vi "MUSIQCTrapControlNoStalling.vi"() -> ()   [LabVIEW 2012]
uses:
  <vilib>/DAQmx/read.llb/DAQmx Read (Counter U32 1Chan 1Samp).vi
  <vilib>/DAQmx/read.llb/DAQmx Read (Counter 1D U32 1Chan NSamp).vi
  <vilib>/DAQmx/create/channels.llb/DAQmx Create Channel (CO-Pulse Generation-Frequency).vi
  <vilib>/DAQmx/configure/timing.llb/DAQmx Timing (Implicit).vi
  <vilib>/DAQmx/create/channels.llb/DAQmx Create Channel (CI-Count Edges).vi
  <vilib>/DAQmx/configure/timing.llb/DAQmx Timing (Sample Clock).vi
  <vilib>/Analysis/baseanly.llb/Mean (DBL).vi
  <vilib>/DAQmx/miscellaneous.llb/DAQmx Fill In Error Info.vi
  <resource>/objmgr/daqmx.rc
  <vilib>/Analysis/NI_AALBase.lvlib
panel:
  in  "UV firing rate 2":dbl=2.0
  out "mean":i32
  in  "X window size":dbl=5.0
  out "Sample Rate":dbl
  out "PMT Counts 2":cluster{i32, u32}(graph)
  in  "Measure Background":bool
  in  "Pockel":bool=TRUE
  in  "Dump Frequency":dbl
  in  "AutoDump":bool
  out "Auto Loading Elapsed Time":dbl
  out "Loading Start Time":timestamp=timestamp(3525114376.279 s since 1904-01-01)
  in  "UV":bool
  in  "1762":bool
  in  "455 LED":bool
  in  "399 Yb Ionizer":bool
  in  "Oven":bool
  in  "Orange":bool=TRUE
  in  "Sample Time":dbl=0.02 format="%0.2f"
  in  "Threshold":u32
  in  "Auto Load":bool
  in  "RF":bool
  in  "Blue":bool=TRUE
  in  "Red":bool=TRUE
  in  "Samples per averaging\nblock red":i32=20 min=1 step=1
  in  "stop":bool
  out "PMT Counts":cluster{i32, u32}(graph)
  # "Trap 2"
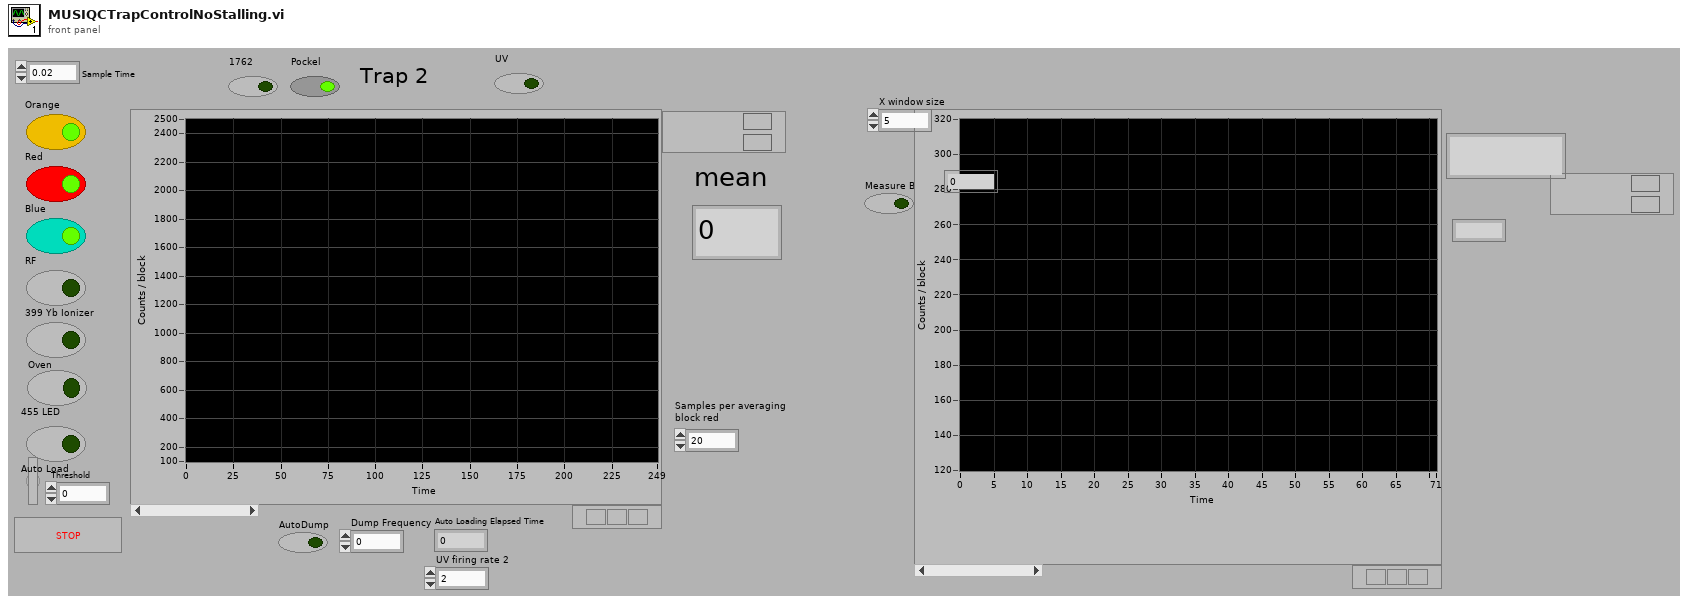
[diagram p1: front panel]
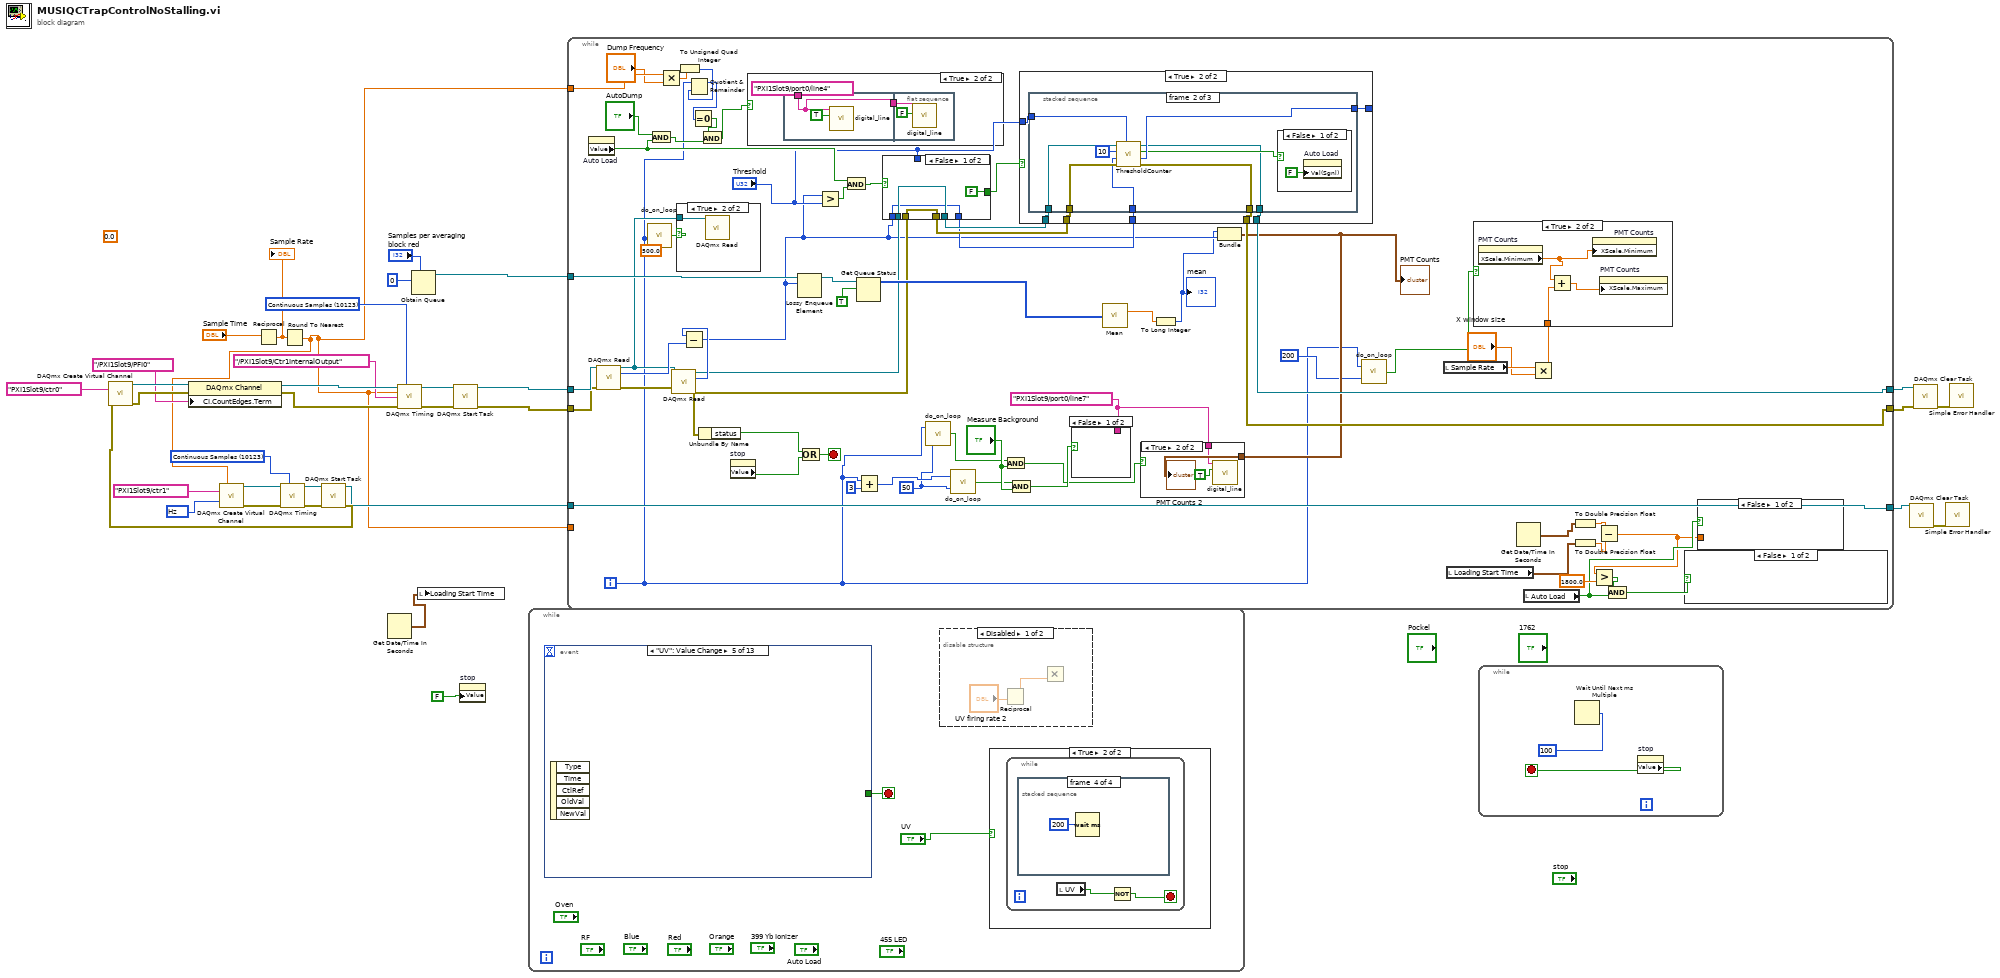
[diagram p0: block diagram]
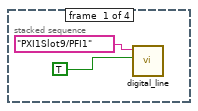
[diagram p3: hidden frame]
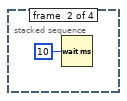
[diagram p4: hidden frame]
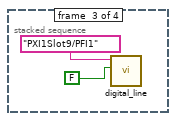
[diagram p5: hidden frame]
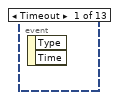
[diagram p7: hidden frame]
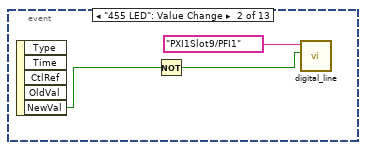
[diagram p8: hidden frame]
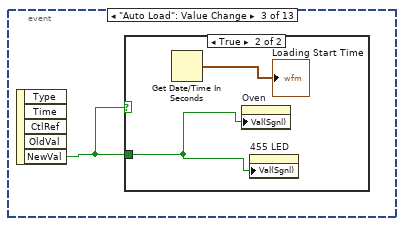
[diagram p9: hidden frame]
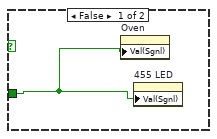
[diagram p10: hidden frame]
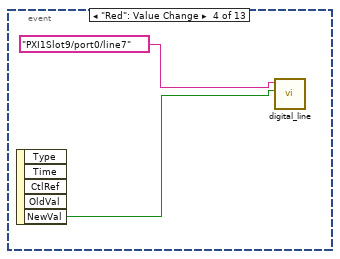
[diagram p11: hidden frame]
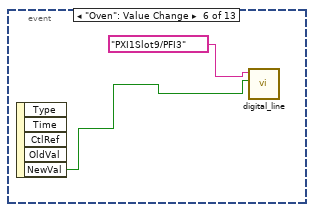
[diagram p12: hidden frame]
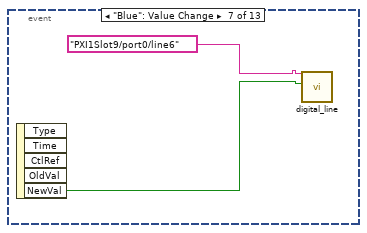
[diagram p13: hidden frame]
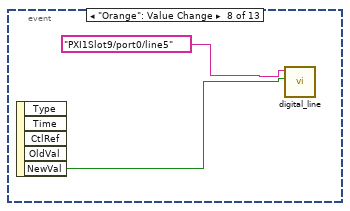
[diagram p14: hidden frame]
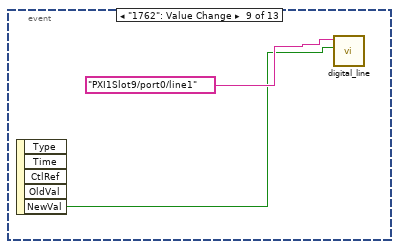
[diagram p15: hidden frame]
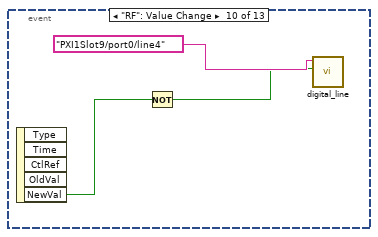
[diagram p16: hidden frame]
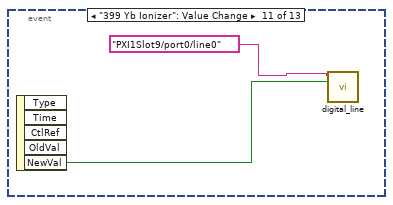
[diagram p17: hidden frame]
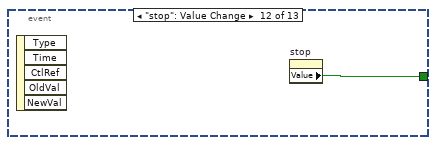
[diagram p18: hidden frame]
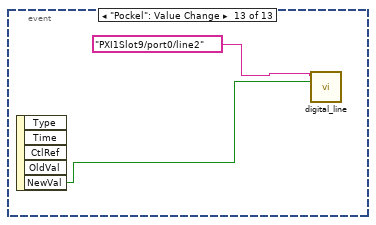
[diagram p19: hidden frame]
diagram:
  (unwired) 0.0 ("x")
  w5 = 10123 items=["Finite Samples"=10178, "Continuous Samples"=10123, "Hardware Timed Single Point"=12522] ("sample mode")
  w12 = 10373 items=["Hz"=10373] ("units")
  w18 = 10123 items=["Finite Samples"=10178, "Continuous Samples"=10123, "Hardware Timed Single Point"=12522] ("sample mode")
  n1 = Reciprocal(x="Sample Time") -> (1/x=w3:dbl)
  "Sample Rate" <- w3
  n2 = Round To Nearest(number=w3) -> (nearest integer value=w2:dbl)
  n3 = call-poly <vilib>:"DAQmx Create Virtual Channel.vi"("frequency"=w2, "counter"=tag "PXI1Slot9/ctr1", "units"=w12) -> ("task out"=w9:refnum<k21>, "error out"=w8:errorcluster)  [unwired: 11 in]
  n4 = call-poly <vilib>:"DAQmx Timing.vi"("task/channels in"=w9, "sample mode"=w5, "error in"=w8) -> ("task out"=w7:refnum<k21>, "error out"=w6:errorcluster)  [unwired: 11 in]
  n5 = call <vilib>:"DAQmx Start Task.vi"("task/channels in"=w7, "error in"=w6) -> ("task out"=w15:refnum<k21>, "error out"=w16:errorcluster)  [unwired: 12 in]
  n6 = call-poly <vilib>:"DAQmx Create Virtual Channel.vi"("counter"=tag "PXI1Slot9/ctr0", "error in"=w16) -> ("task out"=w26:refnum<k21>, "error out"=w25:errorcluster)  [unwired: 12 in]
  n7 = property class="DAQmx Channel"(reference=w26, error in=w25, "CI.CountEdges.Term"=tag "/PXI1Slot9/PFI0") -> (reference out=w28:refnum<k21>, error out=w27:errorcluster)
  n8 = Get Date/Time In Seconds() -> (seconds since 1Jan1904=w4:timestamp)
  n9 = call-poly <vilib>:"DAQmx Timing.vi"("task/channels in"=w28, "sample mode"=w18, "rate"=w2, "source"=tag "/PXI1Slot9/Ctr1InternalOutput", "error in"=w27) -> ("task out"=w33:refnum<k21>, "error out"=w32:errorcluster)  [unwired: 9 in]
  n10 = Obtain Queue(max queue size (-1, unlimited)="Samples per averaging\nblock red", element data type=u32 0) -> (queue out=w21:refnum<queue>)  [unwired: 3 in, 2 out]
  n11 = local write "Loading Start Time"(w4) -> ()
  n12 = call <vilib>:"DAQmx Start Task.vi"("task/channels in"=w33, "error in"=w32) -> ("task out"=w29:refnum<k21>, "error out"=w11:errorcluster)  [unwired: 12 in]
  n13 = property on="stop" class="Bool (strict)"("Value"=FALSE ("stop")) -> ()  [unwired: 2 in, 2 out]
  n14 = while {
    stop <- w36 stop-if-true
    n15 = event shown="[4] \"UV\": Value Change" {
      selector: _ -> [_ _ _ _ _ _ _ _ _ _ _ _ _]
      dyn-events: _ -> [_ _ _ _ _ _ _ _ _ _ _ _ _]
      timeout: _ -> [_ _ _ _ _ _ _ _ _ _ _ _ _]
      tunnel: [_ _ _ _ _ _ _ _ _ _ _ w69 _] -> w36
      event Timeout {
        n16 = event-data() -> ()  [unwired: 1 in, 2 out]
      }
      event "455 LED": Value Change {
        n17 = event-data() -> ("NewVal"=w49:bool)  [unwired: 1 in, 4 out]
        n18 = Not(x=w49) -> (.not. x?=w47:bool)
        n19 = call "digital_line.vi"("Boolean"=w47, "lines"=tag "PXI1Slot9/PFI1") -> ()  [unwired: 5 in, 1 out]
      }
      event "Auto Load": Value Change {
        n20 = event-data() -> ("NewVal"=w50:bool)  [unwired: 1 in, 4 out]
        n21 = case shown="True" w50 {
          tunnel: w50 -> [w51 w52]
          frame False {
            n22 = property on="Oven" class="Bool (strict)"("Val(Sgnl)"=w51) -> ()  [unwired: 2 in, 2 out]
            n23 = property on="455 LED" class="Bool (strict)"("Val(Sgnl)"=w51) -> ()  [unwired: 2 in, 2 out]
          }
          frame True {
            n24 = Get Date/Time In Seconds() -> (seconds since 1Jan1904=→"Loading Start Time":timestamp)
            n25 = property on="Oven" class="Bool (strict)"("Val(Sgnl)"=w52) -> ()  [unwired: 2 in, 2 out]
            n26 = property on="455 LED" class="Bool (strict)"("Val(Sgnl)"=w52) -> ()  [unwired: 2 in, 2 out]
          }
        }
      }
      event "Red": Value Change {
        n27 = event-data() -> ("NewVal"=w54:bool)  [unwired: 1 in, 4 out]
        n28 = call "digital_line.vi"("Boolean"=w54, "lines"=tag "PXI1Slot9/port0/line7") -> ()  [unwired: 5 in, 1 out]
      }
      event "UV": Value Change {
        n29 = event-data() -> ()  [unwired: 1 in, 5 out]
      }
      event "Oven": Value Change {
        n30 = event-data() -> ("NewVal"=w56:bool)  [unwired: 1 in, 4 out]
        n31 = call "digital_line.vi"("Boolean"=w56, "lines"=tag "PXI1Slot9/PFI3") -> ()  [unwired: 5 in, 1 out]
      }
      event "Blue": Value Change {
        n32 = event-data() -> ("NewVal"=w58:bool)  [unwired: 1 in, 4 out]
        n33 = call "digital_line.vi"("Boolean"=w58, "lines"=tag "PXI1Slot9/port0/line6") -> ()  [unwired: 5 in, 1 out]
      }
      event "Orange": Value Change {
        n34 = event-data() -> ("NewVal"=w60:bool)  [unwired: 1 in, 4 out]
        n35 = call "digital_line.vi"("Boolean"=w60, "lines"=tag "PXI1Slot9/port0/line5") -> ()  [unwired: 5 in, 1 out]
      }
      event "1762": Value Change {
        n36 = event-data() -> ("NewVal"=w62:bool)  [unwired: 1 in, 4 out]
        n37 = call "digital_line.vi"("Boolean"=w62, "lines"=tag "PXI1Slot9/port0/line1") -> ()  [unwired: 5 in, 1 out]
      }
      event "RF": Value Change {
        n38 = event-data() -> ("NewVal"=w66:bool)  [unwired: 1 in, 4 out]
        n39 = Not(x=w66) -> (.not. x?=w64:bool)
        n40 = call "digital_line.vi"("Boolean"=w64, "lines"=tag "PXI1Slot9/port0/line4") -> ()  [unwired: 5 in, 1 out]
      }
      event "399 Yb Ionizer": Value Change {
        n41 = event-data() -> ("NewVal"=w67:bool)  [unwired: 1 in, 4 out]
        n42 = call "digital_line.vi"("Boolean"=w67, "lines"=tag "PXI1Slot9/port0/line0") -> ()  [unwired: 5 in, 1 out]
      }
      event "stop": Value Change {
        n43 = event-data() -> ()  [unwired: 1 in, 5 out]
        n44 = property on="stop" class="Bool (strict)"() -> ("Value"=w69:bool)  [unwired: 2 in, 2 out]
      }
      event "Pockel": Value Change {
        n45 = event-data() -> ("NewVal"=w70:bool)  [unwired: 1 in, 4 out]
        n46 = call "digital_line.vi"("Boolean"=w70, "lines"=tag "PXI1Slot9/port0/line2") -> ()  [unwired: 5 in, 1 out]
      }
    }
    n47 = disable-structure shown="Disabled" {
      frame Disabled {
        n48 = Reciprocal(x="UV firing rate 2") -> (1/x=w45:dbl)
        n49 = Multiply(y=w45) -> ()  [unwired: 1 in, 1 out]
      }
      frame Enabled {
      }
    }
    n50 = case shown="True" "UV" {
      frame False {
      }
      frame True {
        n51 = while {
          stop <- w37 stop-if-true
          n52 = stacked-sequence {
            frame #0 {
              n53 = call "digital_line.vi"("Boolean"=TRUE, "lines"=tag "PXI1Slot9/PFI1") -> ()  [unwired: 5 in, 1 out]
            }
            frame #1 {
              n54 = Wait (ms)(milliseconds to wait=u32 10) -> ()  [unwired: 1 out]
            }
            frame #2 {
              n55 = call "digital_line.vi"("Boolean"=FALSE, "lines"=tag "PXI1Slot9/PFI1") -> ()  [unwired: 5 in, 1 out]
            }
            frame #3 {
              n56 = Wait (ms)(milliseconds to wait=u32 200) -> ()  [unwired: 1 out]
            }
          }
          n57 = local read "UV"() -> (w38:bool)
          n58 = Not(x=w38) -> (.not. x?=w37:bool)
        }
      }
    }
  }
  n59 = while {
    tunnel: [w107] -> w31
    tunnel: [w108] -> w30
    tunnel: w29 -> [w134]
    tunnel: w21 -> [w133]
    tunnel: w15 -> [w129]
    tunnel: [w129] -> w13
    tunnel: w11 -> [w128]
    tunnel: w2 -> [_]
    tunnel: w2 -> [w117]
    i -> [w77]
    stop <- w136 stop-if-true
    w96 = tag "PXI1Slot9/port0/line7" ("lines")
    w74 = 50 ("y")
    n60 = property on="Auto Load" class="Bool (strict)"() -> ("Value"=w112:bool)  [unwired: 2 in, 2 out]
    n61 = call-poly <vilib>:"DAQmx Read.vi"("task/channels in"=w134, "error in"=w128) -> ("task out"=w80:refnum<k21>, "data"=w89:u32, "error out"=w86:errorcluster)  [unwired: 11 in]
    n62 = call "do_on_loop.vi"("loopsToSkip"=500.0, "loopIteration"=w77) -> ("x = 0?"=w81:bool)
    n63 = And(x="AutoDump", y=w112) -> (x .and. y?=w110:bool)
    n64 = Multiply(x=w117, y="Dump Frequency") -> (x*y=w115:dbl)
    n65 = call-poly <vilib>:"DAQmx Read.vi"("task/channels in"=w80, "error in"=w86) -> ("task out"=w87:refnum<k21>, "data"=w88:u32, "error out"=w85:errorcluster)  [unwired: 11 in]
    n66 = case shown="True" w81 {
      tunnel: w80 -> [_ w137]
      frame False {
      }
      frame True {
        n67 = call-poly <vilib>:"DAQmx Read.vi"("task/channels in"=w137) -> ()  [unwired: 12 in, 3 out]
      }
    }
    n68 = To Unsigned Quad Integer(1:w115) -> (0:w114:u64)
    n69 = Subtract(x=w88, y=w89) -> (x-y=w83:u32)
    n70 = Quotient & Remainder(x=w77, y=w114) -> (x-y*floor(x/y)=w113:u64)  [unwired: 1 out]
    n71 = Equal To 0?(x=w113) -> (x = 0?=w111:bool)
    n72 = Unbundle By Name(w85) -> ("status"=w135:bool)
    n73 = And(x=w111, y=w110) -> (x .and. y?=w109:bool)
    n74 = property on="stop" class="Bool (strict)"() -> ("Value"=w131:bool)  [unwired: 2 in, 2 out]
    n75 = case shown="True" w109 {
      frame False {
      }
      frame True {
        n76 = flat-sequence {
          tunnel: tag "PXI1Slot9/port0/line4" ("lines") -> [w161]
          tunnel: [w161] -> w158
          tunnel: w158 -> [w163]
          frame #0 {
            n77 = call "digital_line.vi"("Boolean"=TRUE, "lines"=w161) -> ()  [unwired: 5 in, 1 out]
          }
          frame #1 {
            n78 = call "digital_line.vi"("Boolean"=FALSE, "lines"=w163) -> ()  [unwired: 5 in, 1 out]
          }
        }
      }
    }
    n79 = Lossy Enqueue Element(queue=w133, element=w83) -> (queue out=w132:refnum<queue>)  [unwired: 1 in, 3 out]
    n80 = Or(x=w135, y=w131) -> (x .or. y?=w136:bool)
    n81 = Greater?(x=w83, y="Threshold") -> (0:w130:bool)
    n82 = And(x=w112, y=w130) -> (x .and. y?=w106:bool)
    n83 = Get Queue Status(queue=w132, return elements? (F)=TRUE) -> (elements=w90:u32[])  [unwired: 1 in, 7 out]
    n84 = Add(x=w77, y=3) -> (x+y=w75:i32)
    n85 = case shown="False" w106 {
      tunnel: w87 -> [w147 w157]
      tunnel: w85 -> [w148 w156]
      tunnel: [w148 w155] -> w105
      tunnel: [w147 w154] -> w104
      tunnel: w83 -> [w146 _]
      tunnel: [w146 w152] -> w103
      tunnel: [FALSE ("Over Threshold") w151] -> w102
      tunnel: "Threshold" -> [_ w150]
      frame False {
      }
      frame True {
        n86 = call "ThresholdCounter.vi"("Threshold"=w150, "error in"=w156, "number of samples per channel"=10, "task/channels in"=w157) -> ("error out"=w155:errorcluster, "Final Counter"=w152:u32, "Over Threshold"=w151:bool, "task out"=w154:refnum<k21>)  [unwired: 4 in]
      }
    }
    n87 = call "do_on_loop.vi"("loopsToSkip"=w74, "loopIteration"=w77) -> ("x = 0?"=w76:bool)
    n88 = call "do_on_loop.vi"("loopsToSkip"=w74, "loopIteration"=w75) -> ("x = 0?"=w73:bool)
    n89 = And(x=w76, y="Measure Background") -> (x .and. y?=w94:bool)
    n90 = And(x=w73, y="Measure Background") -> (x .and. y?=w95:bool)
    n91 = case shown="True" w102 {
      tunnel: w104 -> [w167 w175]
      tunnel: w105 -> [w168 w174]
      tunnel: [w167 w173] -> w108
      tunnel: [w168 w172] -> w107
      tunnel: "Threshold" -> [_ w171]
      tunnel: w103 -> [w166 w170]
      tunnel: [w166 w169] -> _
      frame False {
      }
      frame True {
        n92 = stacked-sequence {
          tunnel: w175 -> [_ w186 _]
          tunnel: w174 -> [_ w185 _]
          tunnel: [_ w179 _] -> w173
          tunnel: [_ w180 _] -> w172
          tunnel: w171 -> [_ w178 _]
          tunnel: w170 -> [_ w183 _]
          tunnel: [_ w182 _] -> w169
          frame #0 {
            n93 = call "digital_line.vi"("Boolean"=FALSE, "lines"=tag "PXI1Slot9/port0/line7") -> ()  [unwired: 5 in, 1 out]
          }
          frame #1 {
            n94 = call "ThresholdCounter.vi"("Threshold"=w178, "error in"=w185, "Previous Counter"=w183, "number of samples per channel"=10, "task/channels in"=w186) -> ("error out"=w180:errorcluster, "Final Counter"=w182:u32, "Over Threshold"=w181:bool, "task out"=w179:refnum<k21>)  [unwired: 3 in]
            n95 = case shown="False" w181 {
              frame False {
                n96 = property on="Auto Load" class="Bool (strict)"("Val(Sgnl)"=FALSE ("Auto Load")) -> ()  [unwired: 2 in, 2 out]
              }
              frame True {
              }
            }
          }
          frame #2 {
            n97 = call "digital_line.vi"("Boolean"=TRUE, "lines"=tag "PXI1Slot9/port0/line7") -> ()  [unwired: 5 in, 1 out]
          }
        }
      }
    }
    n98 = case shown="False" w95 {
      tunnel: w96 -> [_ w145]
      frame False {
      }
      frame True {
        n99 = call "digital_line.vi"("Boolean"=FALSE, "lines"=w145) -> ()  [unwired: 5 in, 1 out]
      }
    }
    n100 = call-poly <vilib>:"Mean.vi"("X"=w90) -> ("mean"=w84:dbl)  [unwired: 1 out]
    n101 = To Long Integer(number=w84) -> (32bit integer=w72:i32)
    "mean" <- w72
    n102 = Bundle(w72, w83) -> (w97:cluster{i32, u32})  [unwired: 1 in]
    "PMT Counts" <- w97
    n103 = case shown="True" w94 {
      tunnel: w97 -> [_ w142]
      tunnel: w96 -> [_ w141]
      frame False {
      }
      frame True {
        n104 = call "digital_line.vi"("Boolean"=TRUE, "lines"=w141) -> ()  [unwired: 5 in, 1 out]
        "PMT Counts 2" <- w142
      }
    }
    n105 = call "do_on_loop.vi"("loopsToSkip"=200 ("y"), "loopIteration"=w77) -> ("x = 0?"=w78:bool)
    n106 = local read "Sample Rate"() -> (w93:dbl)
    n107 = local read "Loading Start Time"() -> (w123:timestamp)
    n108 = Get Date/Time In Seconds() -> (seconds since 1Jan1904=w126:timestamp)
    n109 = local read "Auto Load"() -> (w120:bool)
    n110 = Multiply(x=w93, y="X window size") -> (x*y=w91:dbl)
    n111 = case shown="True" w78 {
      tunnel: w91 -> [_ w138]
      frame False {
      }
      frame True {
        n112 = property on="PMT Counts" class="WFChart (strict)"() -> ("XScale.Minimum"=w140:dbl)  [unwired: 2 in, 2 out]
        n113 = Add(x=w140, y=w138) -> (x+y=w139:dbl)
        n114 = property on="PMT Counts" class="WFChart (strict)"("XScale.Minimum"=w140) -> ()  [unwired: 2 in, 2 out]
        n115 = property on="PMT Counts" class="WFChart (strict)"("XScale.Maximum"=w139) -> ()  [unwired: 2 in, 2 out]
      }
    }
    n116 = To Double Precision Float(number=w126) -> (double precision float=w124:dbl)
    n117 = To Double Precision Float(number=w123) -> (double precision float=w125:dbl)
    n118 = Subtract(x=w124, y=w125) -> (x-y=w119:dbl)
    n119 = Greater?(x=w119, y=1800.0) -> (0:w122:bool)
    n120 = And(x=w122, y=w120) -> (x .and. y?=w121:bool)
    n121 = case shown="False" w121 {
      frame False {
      }
      frame True {
        n122 = property on="Auto Load" class="Bool (strict)"("Val(Sgnl)"=FALSE ("Value (Signaling)")) -> ()  [unwired: 2 in, 2 out]
      }
    }
    n123 = case shown="False" w120 {
      tunnel: w119 -> [_ w164]
      frame False {
      }
      frame True {
        "Auto Loading Elapsed Time" <- w164
      }
    }
  }
  n124 = while {
    stop <- w190 stop-if-true
    n125 = Wait Until Next ms Multiple(millisecond multiple=u32 100) -> ()  [unwired: 1 out]
    n126 = property on="stop" class="Bool (strict)"() -> ("Value"=w190:bool)  [unwired: 2 in, 2 out]
  }
  n127 = call <vilib>:"DAQmx Clear Task.vi"("task in"=w13) -> ("error out"=w14:errorcluster)  [unwired: 14 in]
  n128 = call <vilib>:"DAQmx Clear Task.vi"("task in"=w30, "error in"=w31) -> ("error out"=w19:errorcluster)  [unwired: 13 in]
  n129 = call <vilib>:"Simple Error Handler.vi"("error in (no error)"=w14) -> ()  [unwired: 4 in, 5 out]
  n130 = call <vilib>:"Simple Error Handler.vi"("error in (no error)"=w19) -> ()  [unwired: 4 in, 5 out]
